vi "数据时间对齐处理.vi"(9 "待对齐时间":timestamp, 10 "对齐参考时间":timestamp, 11 "已对齐时间输入":timestamp) -> (3 "已对齐时间输出":timestamp)   [LabVIEW 2022 SP3, in "斯坦道总氮.lvlib"]
panel:
  out "已排序的数组":timestamp[](array[timestamp])
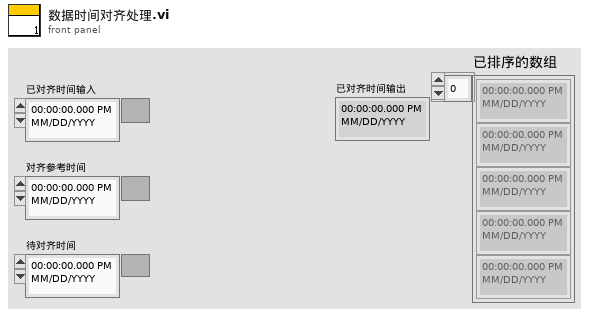
[diagram p1: front panel]
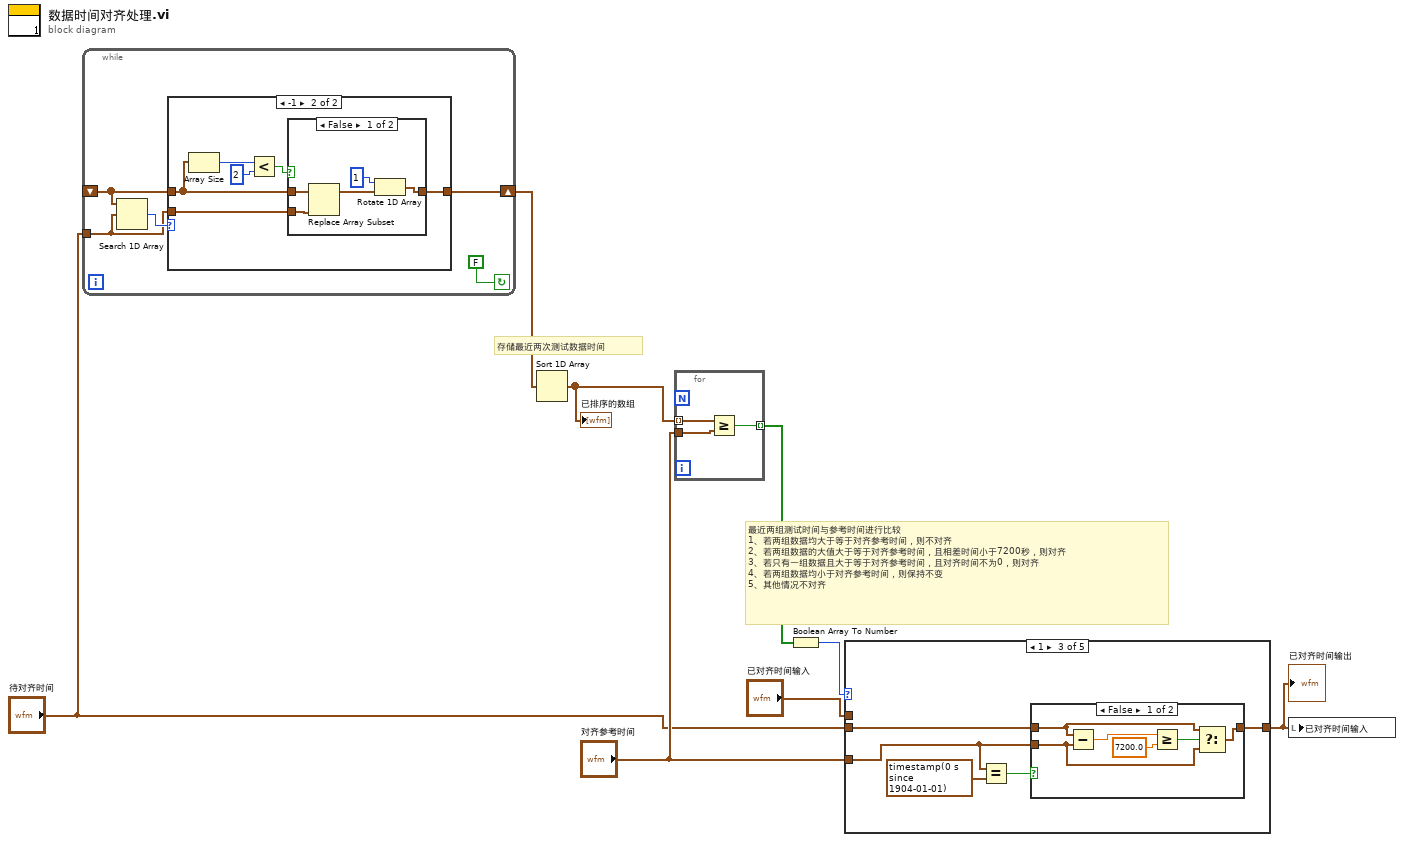
[diagram p0: block diagram]
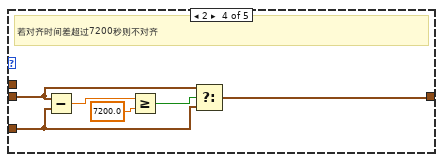
[diagram p5: hidden frame]
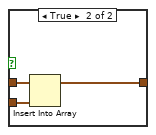
[diagram p8: hidden frame]
diagram:
  # "最近两组测试时间与参考时间进行比较\n1、若两组数据均大于等于对齐参考时间，则不对齐\n2、若两组数据的大值大于等于对齐参考时间，且相差时间小于7200秒，则对齐\n3、若只有一组数据且大于等于对齐参考时间，且对齐时间不为0，则对齐\n4、若两组数据均小于对齐参考时间，则保持不变\n5、其他情况不对齐"
  # "存储最近两次测试数据时间"
  n1 = while {
    shift-right: [w10] -> w3
    shift-left: _ -> [w12]
    tunnel: "待对齐时间" -> [w11]
    stop <- FALSE continue-if-true
    n2 = Search 1D Array(1D array=w12, element=w11) -> (index of element=w13:i32)  [unwired: 1 in]
    n3 = case shown="-1" w13 {
      tunnel: w12 -> [w14 w18]
      tunnel: w11 -> [_ w20]
      tunnel: [w14 w19] -> w10
      frame 0, Default {
      }
      frame -1 {
        n4 = Array Size(array=w18) -> (size(s)=w17:i32)
        n5 = Less?(x=w17, y=2) -> (x < y?=w15:bool)
        n6 = case shown="False" w15 {
          tunnel: w20 -> [w25 w28]
          tunnel: [w21 w27] -> w19
          tunnel: w18 -> [w23 w26]
          frame False {
            n7 = Replace Array Subset(array=w23, new element=w25) -> (w22:timestamp[])  [unwired: 1 in]
            n8 = Rotate 1D Array(1:w22, 2:1 ("n")) -> (0:w21:timestamp[])
          }
          frame True {
            n9 = Insert Into Array(array=w26, new element=w28) -> (w27:timestamp[])  [unwired: 1 in]
          }
        }
      }
    }
  }
  n10 = Sort 1D Array(array=w3) -> (sorted array=w1:timestamp[])
  "已排序的数组" <- w1
  n11 = for {
    tunnel: w1 -> [w31] mode=indexing
    tunnel: "对齐参考时间" -> [w30]
    tunnel: [w29] -> w4 mode=indexing
    n12 = Greater Or Equal?(x=w31, y=w30) -> (x >= y?=w29:bool)
  }
  n13 = Boolean Array To Number(Boolean array=w4) -> (number=w7:u32)
  n14 = case shown="1" w7 {
    tunnel: [w32 w33 w35 w46 w52] -> w2
    tunnel: "待对齐时间" -> [w32 _ w36 w48 w52]
    tunnel: "对齐参考时间" -> [_ _ w34 w47 _]
    tunnel: "已对齐时间输入" -> [_ w33 _ _ _]
    frame Default {
    }
    frame 0 {
    }
    frame 1 {
      n15 = Equal?(x=w34, y=timestamp(0 s since 1904-01-01)) -> (x = y?=w37:bool)
      n16 = case shown="False" w37 {
        tunnel: w36 -> [w41 w45]
        tunnel: [w39 w45] -> w35
        tunnel: w34 -> [w40 _]
        frame False {
          n17 = Subtract(x=w41, y=w40) -> (x-y=w44:dbl)
          n18 = Greater Or Equal?(x=w44, y=7200.0) -> (x >= y?=w42:bool)
          n19 = Select(t=w41, s=w42, f=w40) -> (s? t:f=w39:timestamp)
        }
        frame True {
        }
      }
    }
    frame 2 {
      # "若对齐时间差超过7200秒则不对齐"
      n20 = Subtract(x=w48, y=w47) -> (x-y=w51:dbl)
      n21 = Greater Or Equal?(x=w51, y=7200.0) -> (x >= y?=w49:bool)
      n22 = Select(t=w48, s=w49, f=w47) -> (s? t:f=w46:timestamp)
    }
    frame 3 {
    }
  }
  "已对齐时间输出" <- w2
  n23 = local write "已对齐时间输入"(w2) -> ()
